vi "Async Child.vi"(6 "Alias":string, 7 "Actor in":refnum<class "Actor.lvclass">, 9 "Mid Actors":refnum<class "Actor.lvclass">[](array[class])) -> (0 "Error out":errorcluster, 5 "Actor out":refnum<class "Actor.lvclass">)   [LabVIEW 2020, in "jettl.lvlib" / "Spawn.lvlib"]
uses:
  Spawn.lvlib
  Actor/Actor.lvclass
  Attributes Metadata/Attributes Metadata.lvclass
  Transport/Transport.lvclass
  Msg/Msg.lvclass
  jettl.lvlib
  Msgs.ctl
  Attributes.ctl
  Lifetime.ctl
  Read Self Attributes/Read Self Attributes.lvlib
  Read Self Attributes/Edge Actors.vi
  Read Self Attributes/Core Actors.vi
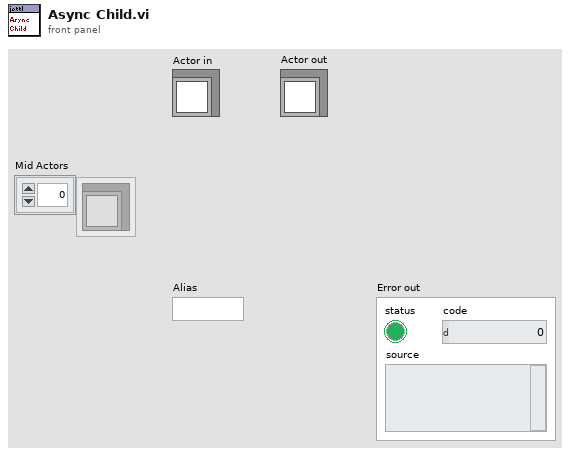
[diagram p1: front panel]
types:
  T1 = typedef "jettl.lvlib/Msgs.ctl" = set{refnum<class "Msg.lvclass">}
  T2 = typedef "jettl.lvlib/Attributes.ctl" = cluster{"Unified Msgs":T1, "Unified Leaf":bool, "Edge Actors":refnum<class "Actor.lvclass">[], "Core Actors":refnum<class "Actor.lvclass">[], "Root":bool, "Alias":string, "UID":i32, "Transport":refnum<class "Transport.lvclass">, "This VI":refnum<vi>, "Attributes Metadata":refnum<class "Attributes Metadata.lvclass">, "Post-Setup Actors":refnum<class "Actor.lvclass">[]}
  T3 = typedef "jettl.lvlib/Lifetime.ctl" = enum16{"Init", "Spawn", "Setup", "Teardown Before Running", "Running", "Stop Called", "Stopping With Children", "Stopping Without Children", "Teardown After Running", "Stopped"}
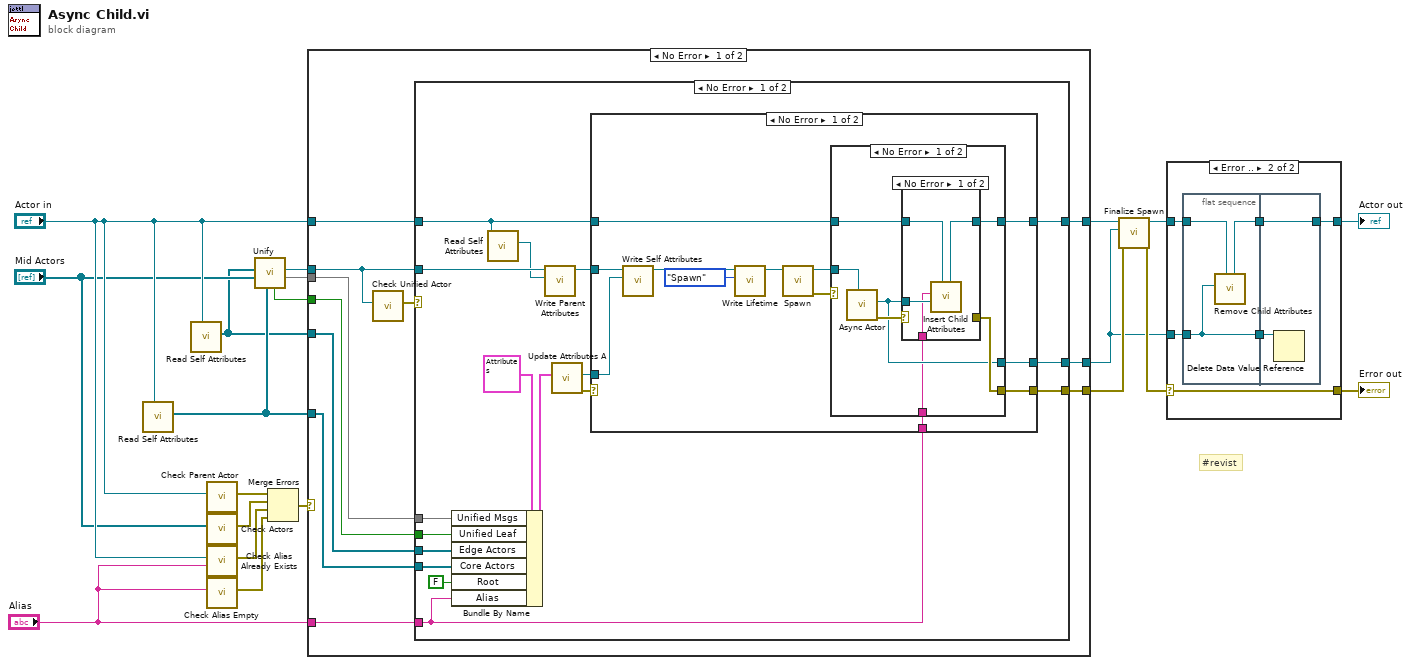
[diagram p0: block diagram]
diagram:
  # "#revist"
  n1 = call-poly "Read Self Attributes.vi"("Actor in"="Actor in") -> ("Core Actors"=w5:refnum<class "Actor.lvclass">[])  [unwired: 10 in]
  n2 = call-poly "Read Self Attributes.vi"("Actor in"="Actor in") -> ("Edge Actors"=w4:refnum<class "Actor.lvclass">[])  [unwired: 10 in]
  n3 = call "Check Parent Actor.vi"("Actor"="Actor in") -> ("Error"=w20:errorcluster)  [unwired: 10 in]
  n4 = call "Check Actors.vi"("Actors"="Mid Actors") -> ("Error"=w13:errorcluster)  [unwired: 10 in]
  n5 = call "Check Alias Already Exists.vi"("Alias"="Alias", "Actor"="Actor in") -> ("Error"=w18:errorcluster)  [unwired: 9 in]
  n6 = call "Check Alias Empty.vi"("Alias"="Alias") -> ("Error"=w17:errorcluster)  [unwired: 10 in]
  n7 = call "Unify.vi"("Core Actors"=w5, "Mid Actors"="Mid Actors", "Edge Actors"=w4) -> ("Unified Msgs"=w3:T1, "Unified Actor"=w2:refnum<class "Actor.lvclass">, "Unified Leaf"=w1:bool)  [unwired: 6 in]
  n8 = Merge Errors(w20, w13, w18, w17) -> (w19:errorcluster)
  n9 = case shown="No Error" w19 {
    selector: w19 -> [_ w80]
    tunnel: "Actor in" -> [w26 w81]
    tunnel: [w31 w80] -> w11
    tunnel: [w30 w81] -> w12
    tunnel: "Alias" -> [w29 _]
    tunnel: [w27 _] -> w8
    tunnel: w5 -> [w25 _]
    tunnel: w4 -> [w24 _]
    tunnel: w3 -> [w23 _]
    tunnel: w2 -> [w21 _]
    tunnel: w1 -> [w22 _]
    frame No Error {
      n10 = call "Check Unified Actor.vi"("Unified Actor"=w21) -> ("Error"=w28:errorcluster)  [unwired: 10 in]
      n11 = case shown="No Error" w28 {
        selector: w28 -> [_ w78]
        tunnel: [w48 w78] -> w31
        tunnel: [w47 w79] -> w30
        tunnel: w26 -> [w35 w79]
        tunnel: w29 -> [w32 _]
        tunnel: w24 -> [w44 _]
        tunnel: w25 -> [w43 _]
        tunnel: w23 -> [w42 _]
        tunnel: w21 -> [w38 _]
        tunnel: w22 -> [w41 _]
        tunnel: [w40 _] -> w27
        frame No Error {
          n12 = Bundle By Name(cluster=T2 {"Unified Msgs"={}, "Unified Leaf"=FALSE, "Edge Actors"=[], "Core Actors"=[], "Root"=FALSE, "Alias"="", "UID"=0, "Transport"=refnum, "This VI"=refnum, "Attributes Metadata"=refnum, "Post-Setup Actors"=[]} ("Attributes"), "Unified Msgs"=w42, "Unified Leaf"=w41, "Edge Actors"=w44, "Core Actors"=w43, "Root"=FALSE, "Alias"=w32) -> (w36:T2)
          n13 = call-dynamic "Read Self Attributes.vi"("Actor in"=w35) -> ("Self Attributes"=w34:refnum<data-value>)  [unwired: 10 in]
          n14 = call-dynamic "Write Parent Attributes.vi"("Parent Attributes"=w34, "Actor in"=w38) -> ("Actor out"=w37:refnum<class "Actor.lvclass">)  [unwired: 9 in]
          n15 = call "Update Attributes A.vi"("Attributes"=w36) -> ("Error out"=w33:errorcluster, "Attributes out"=w39:refnum<data-value>)  [unwired: 9 in]
          n16 = case shown="No Error" w33 {
            selector: w33 -> [_ w77]
            tunnel: [w60 w77] -> w48
            tunnel: [w59 w76] -> w47
            tunnel: [w53 _] -> w40
            tunnel: w39 -> [w52 _]
            tunnel: w37 -> [w51 _]
            tunnel: w35 -> [w50 w76]
            tunnel: w32 -> [w49 _]
            frame No Error {
              n17 = call-dynamic "Write Self Attributes.vi"("Self Attributes"=w52, "Actor in"=w51) -> ("Actor out"=w56:refnum<class "Actor.lvclass">)  [unwired: 9 in]
              n18 = call-dynamic "Write Lifetime.vi"("Lifetime"=Lifetime."Spawn", "Actor in"=w56) -> ("Actor out"=w55:refnum<class "Actor.lvclass">)  [unwired: 9 in]
              n19 = call-dynamic "Spawn.vi"("Actor in"=w55) -> ("Error out"=w54:errorcluster, "Actor out"=w58:refnum<class "Actor.lvclass">)  [unwired: 9 in]
              n20 = case shown="No Error" w54 {
                selector: w54 -> [_ w74]
                tunnel: [w67 w74] -> w60
                tunnel: [w66 w75] -> w59
                tunnel: w50 -> [w65 w75]
                tunnel: w58 -> [w63 _]
                tunnel: [w62 _] -> w53
                tunnel: w49 -> [w61 _]
                frame No Error {
                  n21 = call "Async Actor.vi"("Actor in"=w63) -> ("Error out"=w64:errorcluster, "Attributes"=w62:refnum<data-value>)  [unwired: 9 in]
                  n22 = case shown="No Error" w64 {
                    selector: w64 -> [_ w72]
                    tunnel: w65 -> [w71 w73]
                    tunnel: [w70 w73] -> w66
                    tunnel: w62 -> [w69 _]
                    tunnel: [_ w72] -> w67
                    tunnel: w61 -> [w68 _]
                    frame No Error {
                      n23 = call "Insert Child Attributes.vi"("Actor in"=w71, "Child Attributes"=w69, "Alias"=w68) -> ("Actor out"=w70:refnum<class "Actor.lvclass">)  [unwired: 8 in]
                    }
                    frame Error {
                    }
                  }
                }
                frame Error {
                }
              }
            }
            frame Error {
            }
          }
        }
        frame Error {
        }
      }
    }
    frame Error {
    }
  }
  n24 = call-dynamic "Finalize Spawn.vi"("Error in"=w11, "Attributes"=w8, "Actor in"=w12) -> ("Error out"=w10:errorcluster, "Actor out"=w6:refnum<class "Actor.lvclass">)  [unwired: 7 in]
  n25 = case shown="Error .." w10 {
    selector: w10 -> [_ w88]
    tunnel: [_ w88] -> w9
    tunnel: w8 -> [_ w87]
    tunnel: [w82 w84] -> w7
    tunnel: w6 -> [w82 w85]
    frame No Error {
    }
    frame Error {
      n26 = flat-sequence {
        tunnel: w87 -> [w90]
        tunnel: [w90] -> w86
        tunnel: w85 -> [w91]
        tunnel: [w89] -> w83
        tunnel: w86 -> [w93]
        tunnel: [w92] -> w84
        tunnel: w83 -> [w92]
        frame #0 {
          n27 = call "Remove Child Attributes.vi"("Actor in"=w91, "Child Attributes"=w90) -> ("Actor out"=w89:refnum<class "Actor.lvclass">)  [unwired: 9 in]
        }
        frame #1 {
          n28 = Delete Data Value Reference(data value reference=w93) -> ()  [unwired: 1 in, 2 out]
        }
      }
    }
  }
  "Actor out" <- w7
  "Error out" <- w9
